vi "Panel.vi"(11 "TipPanel in":refnum<class "TipPanel.lvclass">) -> ()   [LabVIEW 2021, in "TipStripOOPanel.lvlib" / "TipPanel.lvclass"]
uses:
  TipPanel.lvclass
  <vilib>/IlluminatedG/IG OOPanel/OOPanel/Panel/Panel.lvclass
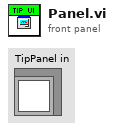
[diagram p1: front panel]
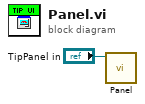
[diagram p0: block diagram]
diagram:
  n1 = call-parent "Panel.vi"("Panel in"="TipPanel in") -> ()  [unwired: 11 in]
